vi "moveAndMeasureAngle.vi"() -> ()   [LabVIEW 2022 SP3]
uses:
  <vilib>/MakerHub/LINX/Public/Utilities/Open Serial.vi
  <vilib>/MakerHub/LINX/Public/Sensors/Motion/Servo/Servo Open N Channels.vi
  <vilib>/addons/control/pid/pid.llb/PID (DBL).vi
  <vilib>/MakerHub/LINX/Public/Sensors/Motion/Servo/Servo Set Pulse Width N Channels.vi
  <vilib>/MakerHub/LINX/Public/Sensors/Motion/Servo/Servo Close N Channels.vi
  <vilib>/MakerHub/LINX/LMH-LINX.lvlib
  <vilib>/MakerHub/LINX/Public/Sensors/Motion/Servo/Servo.lvlib
  <vilib>/addons/control/pid/NI_PID_pid.lvlib
panel:
  in  "PID gains Pitch":T1={"proportional gain (Kc)"=1.0, "integral time (Ti, min)"=0.01, "derivative time (Td, min)"=0.0} {"derivative time (Td, min)" format="%.3f"; "integral time (Ti, min)" format="%.3f"; "proportional gain (Kc)" format="%.3f"}
  in  "PID gains Yaw":T1={"proportional gain (Kc)"=1.0, "integral time (Ti, min)"=0.01, "derivative time (Td, min)"=0.0} {"derivative time (Td, min)" format="%.3f"; "integral time (Ti, min)" format="%.3f"; "proportional gain (Kc)" format="%.3f"}
  out "pitch fixed":dbl
  out "yaw fixed":dbl
  in  "Lock Button":bool
  out "roll":dbl
  out "pitch":dbl
  out "yaw":dbl
  in  "Left":bool
  in  "Right":bool
  in  "Down":bool
  in  "Up":bool
  in  "stop 2":bool
  out "String":string="test"
  in  "Serial Port":refnum<visa-resource-name>="N/A"
  in  "stop":bool
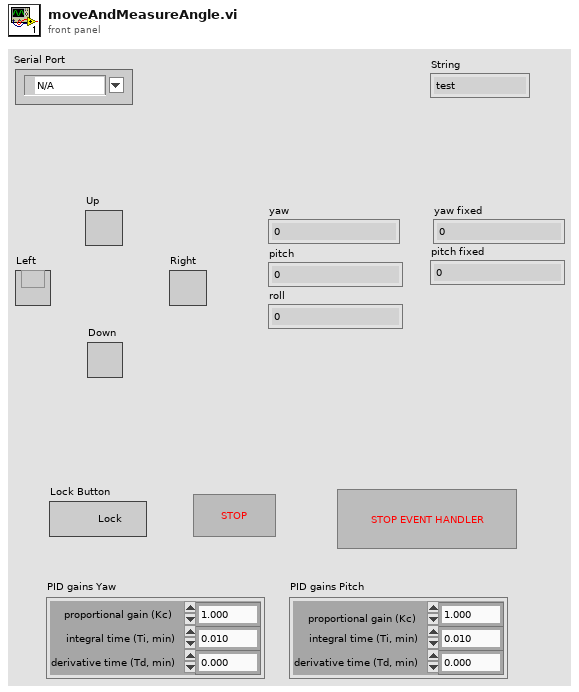
[diagram p1: front panel]
types:
  T1 = cluster{"proportional gain (Kc)":dbl, "integral time (Ti, min)":dbl, "derivative time (Td, min)":dbl}
  T2 = typedef "LMH-LINX.lvlib/LINX Ref.ctl" = cluster{"IO":T3, "Interface":T4, "LINX Device Config":T5}
  T3 = typedef "LMH-LINX.lvlib/Platform.ctl" = enum16{"Remote", "Local"}
  T4 = typedef "LMH-LINX.lvlib/Interface.ctl" = enum16{"Serial", "TCP"}
  T5 = typedef "LMH-LINX.lvlib/Device.lvlib/LINX Device Config.ctl" = cluster{"Interface":T4, "COM Port":refnum<visa-resource-name>, "TCP Configuration":T6, "Device Family":u8, "Device ID":u8, "Device Name":string, "TCP Ref":refnum<k5>, "Channels":T7}
  T6 = typedef "LMH-LINX.lvlib/Device.lvlib/TCP Config.ctl" = cluster{"IP Address":string, "Port":u16}
  T7 = typedef "LMH-LINX.lvlib/Channels.ctl" = cluster{"DI":u8[], "DO":u8[], "AI":u8[], "AO":u8[], "PWM":u8[], "QE":u8[], "UART":u8[], "I2C 2":u8[], "SPI":u8[], "CAN":u8[], "Servo":u8[], "AI Ref (V)":dbl, "AI Resolution (Bits)":u8, "AO Ref (V)":dbl, "AO Resolution (Bits)":u8}
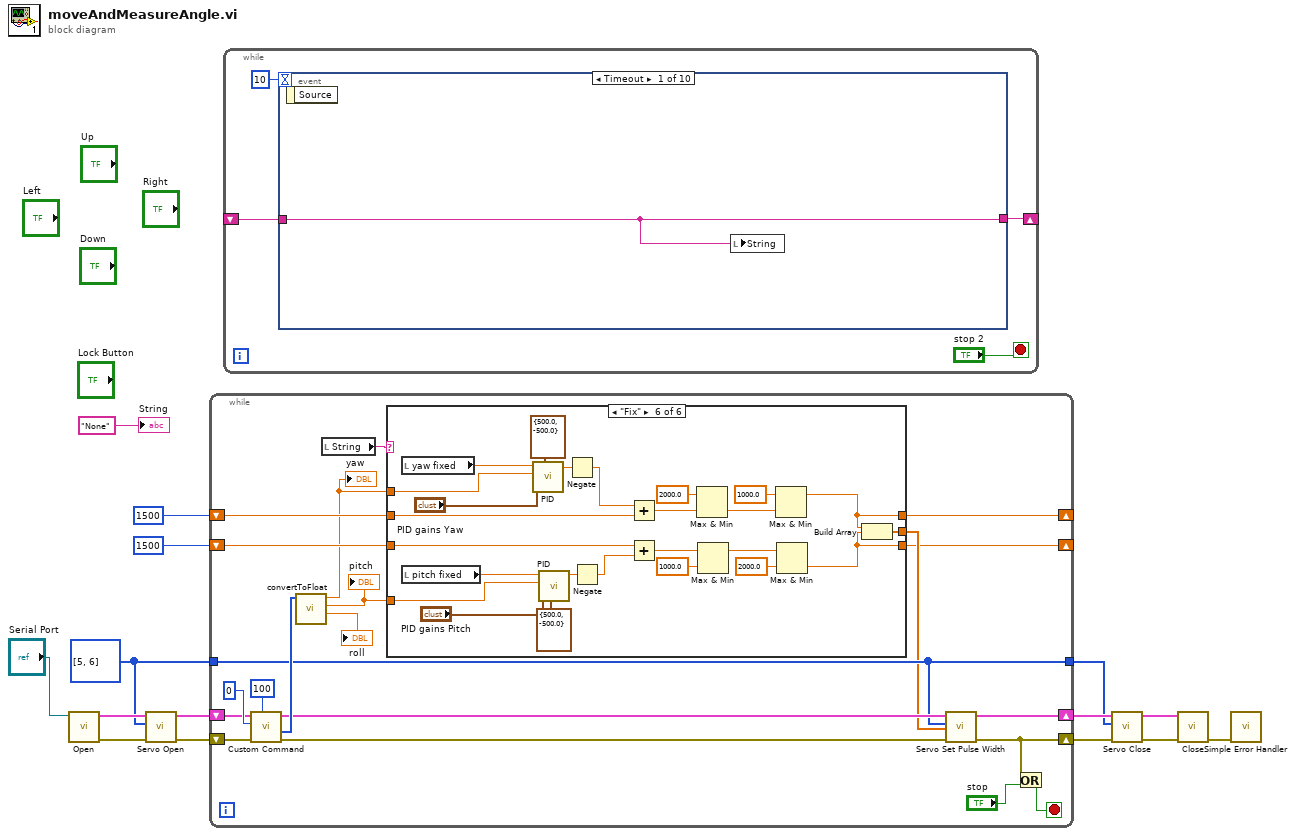
[diagram p0: block diagram]
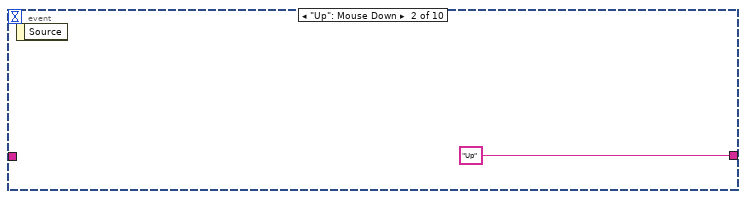
[diagram p2: hidden frame]
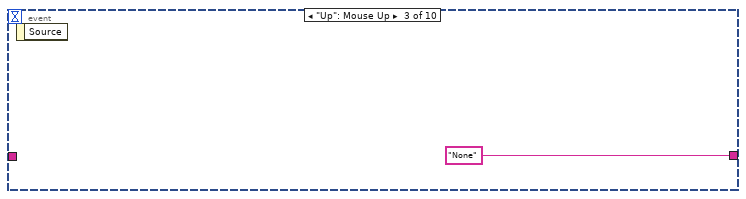
[diagram p3: hidden frame]
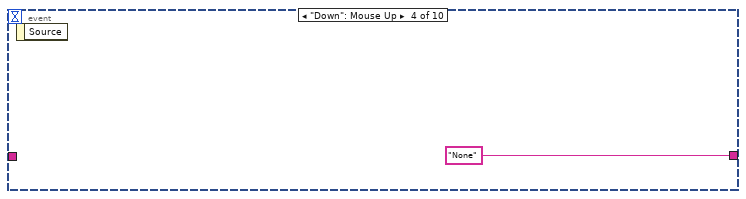
[diagram p4: hidden frame]
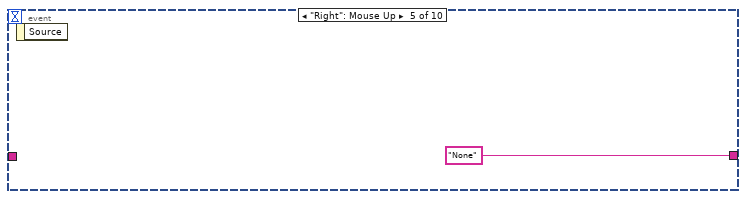
[diagram p5: hidden frame]
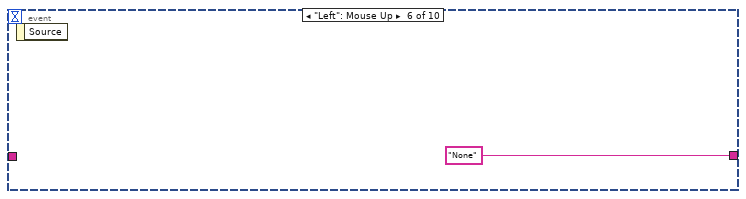
[diagram p6: hidden frame]
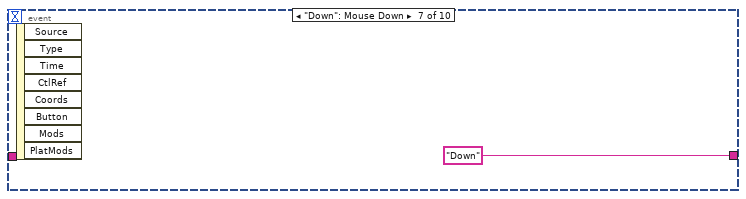
[diagram p7: hidden frame]
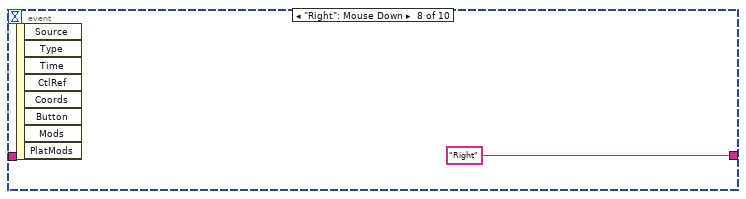
[diagram p8: hidden frame]
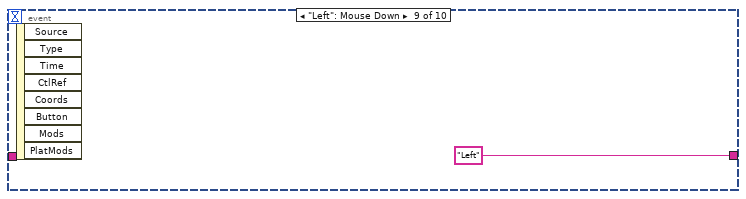
[diagram p9: hidden frame]
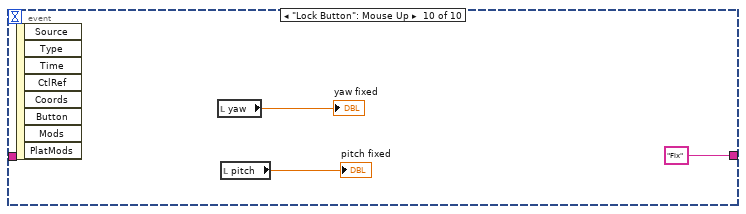
[diagram p10: hidden frame]
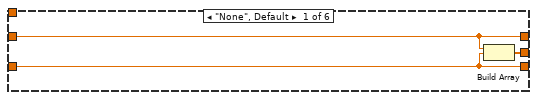
[diagram p11: hidden frame]
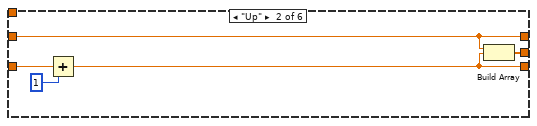
[diagram p12: hidden frame]
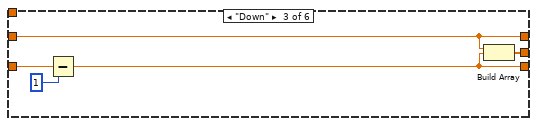
[diagram p13: hidden frame]
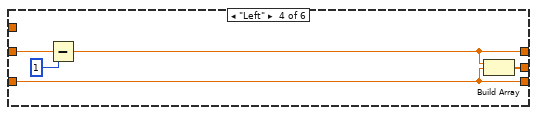
[diagram p14: hidden frame]
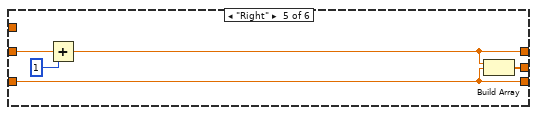
[diagram p15: hidden frame]
diagram:
  w6 = u8[] [5, 6] ("Servo Channels")
  n1 = call-poly <vilib>:"Open.vi"("Serial Port"="Serial Port") -> ("Error Out"=w14:errorcluster, "LINX Resource"=w15:T2)  [unwired: 8 in, 1 out]
  n2 = call-poly <vilib>:"Servo Open.vi"("Error In"=w14, "Servo Channels"=w6, "LINX Resource"=w15) -> ("Error Out"=w12:errorcluster, "LINX Resource"=w13:T2)  [unwired: 7 in]
  n3 = while {
    shift-right: [w29] -> w11
    shift-left: w13 -> [w33]
    shift-right: [w26] -> w10
    shift-left: w12 -> [w32]
    tunnel: w6 -> [w25]
    tunnel: [w25] -> w5
    shift-right: [w19] -> _
    shift-left: 1500 -> [w23]
    shift-right: [w20] -> _
    shift-left: 1500 -> [w22]
    stop <- w28 stop-if-true
    n4 = call <vilib>:"Custom Command.vi"("Timeout (100 ms)"=100, "Error In"=w32, "Custom Command Number"=u16 0, "LINX Resource"=w33) -> ("Error Out"=w30:errorcluster, "Response"=w34:u8[], "LINX Resource"=w31:T2)  [unwired: 4 in, 1 out]
    n5 = call "convertToFloat.vi"("Response"=w34) -> ("roll"=→"roll":dbl, "pitch"=w16:dbl, "yaw"=w17:dbl)  [unwired: 8 in]
    "yaw" <- w17
    "pitch" <- w16
    n6 = local read "String"() -> (w24:string)
    n7 = case shown="\"Fix\"" w24 {
      tunnel: w23 -> [w38 w43 w48 w51 w56 w75]
      tunnel: w22 -> [w37 w41 w46 w52 w57 w74]
      tunnel: [w39 w44 w49 w54 w59 w84] -> w21
      tunnel: [w37 w42 w47 w52 w57 w64] -> w20
      tunnel: [w38 w43 w48 w50 w55 w69] -> w19
      tunnel: w17 -> [_ _ _ _ _ w82]
      tunnel: w16 -> [_ _ _ _ _ w78]
      frame "None", Default {
        n8 = Build Array(w38, w37) -> (w39:dbl[])
      }
      frame "Up" {
        n9 = Add(x=w41, y=1) -> (x+y=w42:dbl)
        n10 = Build Array(w43, w42) -> (w44:dbl[])
      }
      frame "Down" {
        n11 = Subtract(x=w46, y=1) -> (x-y=w47:dbl)
        n12 = Build Array(w48, w47) -> (w49:dbl[])
      }
      frame "Left" {
        n13 = Subtract(x=w51, y=1) -> (x-y=w50:dbl)
        n14 = Build Array(w50, w52) -> (w54:dbl[])
      }
      frame "Right" {
        n15 = Add(x=w56, y=1) -> (x+y=w55:dbl)
        n16 = Build Array(w55, w57) -> (w59:dbl[])
      }
      frame "Fix" {
        n17 = local read "yaw fixed"() -> (w83:dbl)
        n18 = local read "pitch fixed"() -> (w79:dbl)
        n19 = call-poly <vilib>:"PID.vi"("output range"=cluster{"output high":dbl, "output low":dbl} {"output high"=500.0, "output low"=-500.0}, "PID gains"="PID gains Yaw", "process variable"=w82, "setpoint"=w83) -> ("output"=w62:dbl)  [unwired: 6 in, 1 out]
        n20 = call-poly <vilib>:"PID.vi"("output range"=cluster{"output high":dbl, "output low":dbl} {"output high"=500.0, "output low"=-500.0}, "PID gains"="PID gains Pitch", "process variable"=w78, "setpoint"=w79) -> ("output"=w60:dbl)  [unwired: 6 in, 1 out]
        n21 = Negate(x=w62) -> (-x=w63:dbl)
        n22 = Negate(x=w60) -> (-x=w61:dbl)
        n23 = Add(x=w63, y=w75) -> (x+y=w73:dbl)
        n24 = Add(x=w74, y=w61) -> (x+y=w68:dbl)
        n25 = Max & Min(x=2000.0, y=w73) -> (min(x,y)=w71:dbl)  [unwired: 1 out]
        n26 = Max & Min(x=w68, y=1000.0) -> (max(x,y)=w66:dbl)  [unwired: 1 out]
        n27 = Max & Min(x=1000.0, y=w71) -> (max(x,y)=w69:dbl)  [unwired: 1 out]
        n28 = Max & Min(x=w66, y=2000.0) -> (min(x,y)=w64:dbl)  [unwired: 1 out]
        n29 = Build Array(w69, w64) -> (w84:dbl[])
      }
    }
    n30 = call-poly <vilib>:"Servo Set Pulse Width.vi"("Error In"=w30, "Pulse Widths (uS)"=w21, "Servo Channels"=w25, "LINX Resource"=w31) -> ("Error Out"=w26:errorcluster, "LINX Resource"=w29:T2)  [unwired: 6 in]
    n31 = Or(x=w26, y="stop") -> (x .or. y?=w28:bool)
  }
  n32 = while {
    shift-right: [w86] -> _
    shift-left: _ -> [w85]
    stop <- "stop 2" stop-if-true
    n33 = event shown="[0] Timeout" {
      selector: _ -> [_ _ _ _ _ _ _ _ _ _]
      dyn-events: _ -> [_ _ _ _ _ _ _ _ _ _]
      timeout: 10 -> [_ _ _ _ _ _ _ _ _ _]
      tunnel: [w89 "Up" ("String") "None" ("String") "None" ("String") "None" ("String") "None" ("String") "Down" ("String") "Right" ("String") "Left" ("String") "Fix" ("String")] -> w86
      tunnel: w85 -> [w89 _ _ _ _ _ _ _ _ _]
      event Timeout {
        n34 = event-data() -> ()  [unwired: 1 in, 1 out]
        n35 = local write "String"(w89) -> ()
      }
      event "Up": Mouse Down {
        n36 = event-data() -> ()  [unwired: 1 in, 1 out]
      }
      event "Up": Mouse Up {
        n37 = event-data() -> ()  [unwired: 1 in, 1 out]
      }
      event "Down": Mouse Up {
        n38 = event-data() -> ()  [unwired: 1 in, 1 out]
      }
      event "Right": Mouse Up {
        n39 = event-data() -> ()  [unwired: 1 in, 1 out]
      }
      event "Left": Mouse Up {
        n40 = event-data() -> ()  [unwired: 1 in, 1 out]
      }
      event "Down": Mouse Down {
        n41 = event-data() -> ()  [unwired: 1 in, 8 out]
      }
      event "Right": Mouse Down {
        n42 = event-data() -> ()  [unwired: 1 in, 8 out]
      }
      event "Left": Mouse Down {
        n43 = event-data() -> ()  [unwired: 1 in, 8 out]
      }
      event "Lock Button": Mouse Up {
        n44 = event-data() -> ()  [unwired: 1 in, 8 out]
        n45 = local read "yaw"() -> (→"yaw fixed":dbl)
        n46 = local read "pitch"() -> (→"pitch fixed":dbl)
      }
    }
  }
  n47 = call-poly <vilib>:"Servo Close.vi"("Error In"=w10, "Servo Channels"=w5, "LINX Resource"=w11) -> ("Error Out"=w8:errorcluster, "LINX Resource"=w9:T2)  [unwired: 7 in]
  n48 = call <vilib>:"Close.vi"("Error In"=w8, "LINX Resource"=w9) -> ("Error Out"=w4:errorcluster)  [unwired: 9 in]
  n49 = call <vilib>:"Simple Error Handler.vi"("error in (no error)"=w4) -> ()  [unwired: 4 in, 5 out]
  "String" <- "None" ("String")
